vi "Invalid Response.vi"(7 "error source vi name":string, 8 "error in (no error)":errorcluster, 9 "actual response":string, 10 "expected response":string, 11 "Interface in":refnum<class "Interface.lvclass">) -> (0 "error out":errorcluster, 3 "Interface out":refnum<class "Interface.lvclass">)   [LabVIEW 2017, in "DSF Core.lvlib" / "Interface.lvclass"]
uses:
  Interface/Interface.lvclass
  Interface/Errors.ctl
  LabVIEW-Memory/Source/Static Error Handling.lvlib
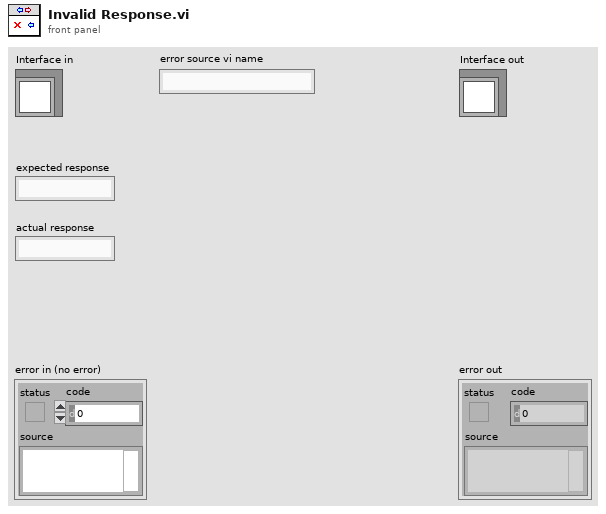
[diagram p1: front panel]
types:
  T1 = typedef "DSF Core.lvlib/Interface.lvclass/Errors.ctl" = enum16{"Command Timeout", "Response Timeout", "Error Timeout", "Invalid Response", "Invalid Response Parameters"}
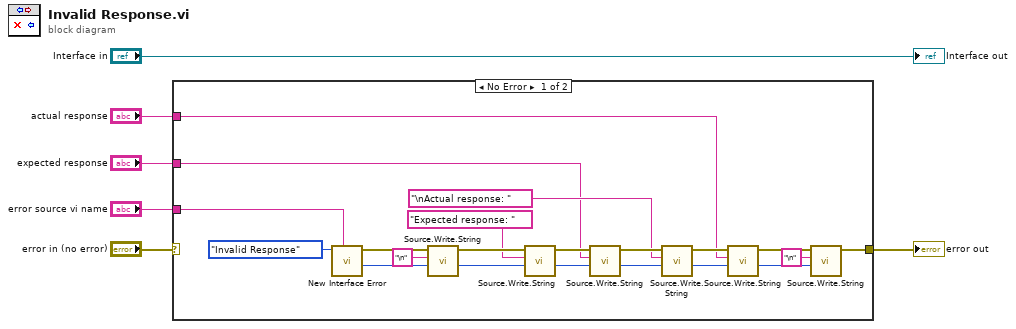
[diagram p0: block diagram]
diagram:
  n1 = case shown="No Error" "error in (no error)" {
    selector: "error in (no error)" -> [_ w28]
    tunnel: [w10 w28] -> w4
    tunnel: "error source vi name" -> [w27 _]
    tunnel: "actual response" -> [w9 _]
    tunnel: "expected response" -> [w8 _]
    frame No Error {
      n2 = call "New Interface Error.vi"("error source vi name"=w27, "error"=Errors."Invalid Response") -> ("new offset"=w25:i32, "error out"=w26:errorcluster)  [unwired: 8 in]
      n3 = call "Source.Write.String.vi"("offset"=w25, "string"="\n", "error in"=w26) -> ("new offset"=w22:i32, "error out"=w23:errorcluster)  [unwired: 7 in]
      n4 = call "Source.Write.String.vi"("offset"=w22, "string"="Expected response: ", "error in"=w23) -> ("new offset"=w21:i32, "error out"=w20:errorcluster)  [unwired: 7 in]
      n5 = call "Source.Write.String.vi"("offset"=w21, "string"=w8, "error in"=w20) -> ("new offset"=w17:i32, "error out"=w18:errorcluster)  [unwired: 7 in]
      n6 = call "Source.Write.String.vi"("offset"=w17, "string"="\nActual response: ", "error in"=w18) -> ("new offset"=w14:i32, "error out"=w15:errorcluster)  [unwired: 7 in]
      n7 = call "Source.Write.String.vi"("offset"=w14, "string"=w9, "error in"=w15) -> ("new offset"=w12:i32, "error out"=w13:errorcluster)  [unwired: 7 in]
      n8 = call "Source.Write.String.vi"("offset"=w12, "string"="\n", "error in"=w13) -> ("error out"=w10:errorcluster)  [unwired: 7 in, 1 out]
    }
    frame Error {
    }
  }
  "error out" <- w4
  "Interface out" <- "Interface in"
